vi "UI Example Subpanel.vi"(11 "CIF_UI in":refnum<class "CIF_UI.lvclass">) -> ()   [LabVIEW 2021, in "CIF Manager UI.lvlib"]
uses:
  CIF Manager UI.lvlib
  CIFUI/CIF_UI.lvclass
  CIFUI/Typedef/Core UI References.ctl
  CIFCore/Grpc/CIFCoreWrapper/CIFCoreWrapper.lvlib
panel:
  out "Current Config":string
  in  "New Config":string
  in  "Update Config":bool
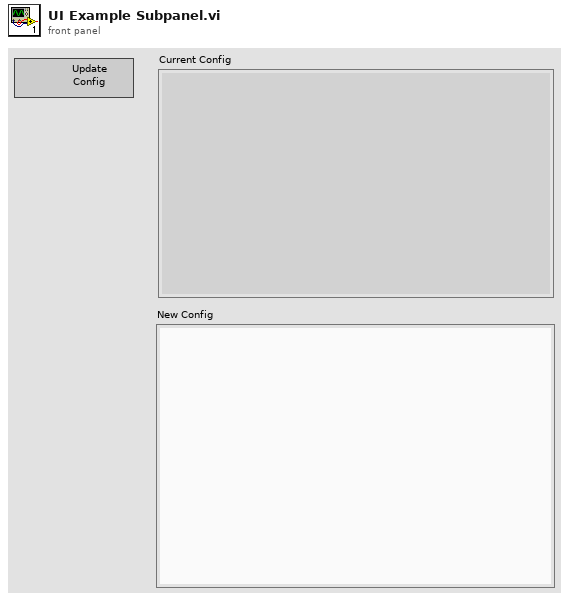
[diagram p1: front panel]
types:
  T1 = typedef "CIF_UI.lvclass/Core UI References.ctl" = cluster{"Discovered Plugins":refnum<vi>, "Discovered Plugins Valid":bool, "Loaded Plugins":refnum<vi>, "Loaded Plugins Valid":bool, "Publisher Channels":refnum<vi>, "Publisher Channels Valid":bool, "Subscriber Channels":refnum<vi>, "Subscriber Channels Valid":bool, "Plugin Status":refnum<vi>, "Plugin Status Valid":bool, "Channel Connection":refnum<vi>, "Channel Connection Valid":bool, "New Plugin Load":refnum<vi>, "New Plugin Load Valid":bool, "Errors":refnum<vi>, "Errors Valid":bool, "Plugin to Abort":refnum<vi>, "Plugin to Abort Valid":bool, "Connection":refnum<vi>, "Connection Valid":bool, "Exit":refnum<vi>, "Exit Valid":bool, "Run Listen":refnum<vi>, "Run Listen Valid":bool, "CIF Manager Tab":refnum<vi>, "Manger Tab Valid":bool, "Clear Local Error":refnum<vi>, "Clear Local Error Valid":bool, "Local Error":refnum<vi>, "Local Error Valid":bool, "System Errors":refnum<vi>, "System Errors Valid":bool, "Plugin Selection":refnum<vi>, "Plugin Selection Valid":bool}
  T2 = typedef "CIF_UI.lvclass/Plugin Connections.ctl" = cluster{"gRPC ID":T3, "Plugin Info":T4}
  T3 = typedef "grpc-lvsupport-release.lvlib/grpcId.ctl" = u64
  T4 = typedef "CIF_UI.lvclass/PluginInfo.ctl" = cluster{"Name":string, "Type":string, "grpc_port":i32, "Version":T5, "Node Status":T6}
  T5 = typedef "CIF_UI.lvclass/Version.ctl" = cluster{"Major":i32, "Minor":i32, "Fix":i32}
  T6 = typedef "CIFCoreCommon.lvlib/gRPC Reported Plugin Status.ctl" = cluster{"State":T7, "Timing Statistics (us)":T8, "FIFO Statistics (us)":T10, "error":T11, "Monitor Doubles":T12, "Monitor U64":T13, "Monitor I64":T14}
  T7 = typedef "CIFCoreCommon.lvlib/Plugin State.ctl" = enum32{"Null", "Creating", "Listening", "Running", "CleaningUp", "Destroying"}
  T8 = typedef "CIFCoreCommon.lvlib/Timing Statistics.ctl" = cluster{"Period":T9, "Wake Error":T9, "Execute":T9, "Housekeep":T9, "Idle":T9, "Cleanup":T9, "Custom 1 (custom units)":T9, "Custom 2 (custom units)":T9}
  T9 = typedef "CIFCoreCommon.lvlib/Timing Stats Base.ctl" = cluster{"Max":i64, "Avg":dbl, "Min":i64}
  T10 = typedef "CIFCoreCommon.lvlib/FIFO Statistics.ctl" = cluster{"From T0":T9, "From Previous Plugin":T9, "Output Error":T9}
  T11 = typedef "CIFCoreCommon.lvlib/Simple Error.ctl" = cluster{"status":bool, "code":i32}
  T12 = typedef "CIFCoreCommon.lvlib/Monitor Doubles.ctl" = cluster{"1":dbl, "2":dbl, "3":dbl, "4":dbl}
  T13 = typedef "CIFCoreCommon.lvlib/Monitor U64.ctl" = cluster{"1":u64, "2":u64, "3":u64, "4":u64}
  T14 = typedef "CIFCoreCommon.lvlib/Monitor I64.ctl" = cluster{"1":i64, "2":i64, "3":i64, "4":i64}
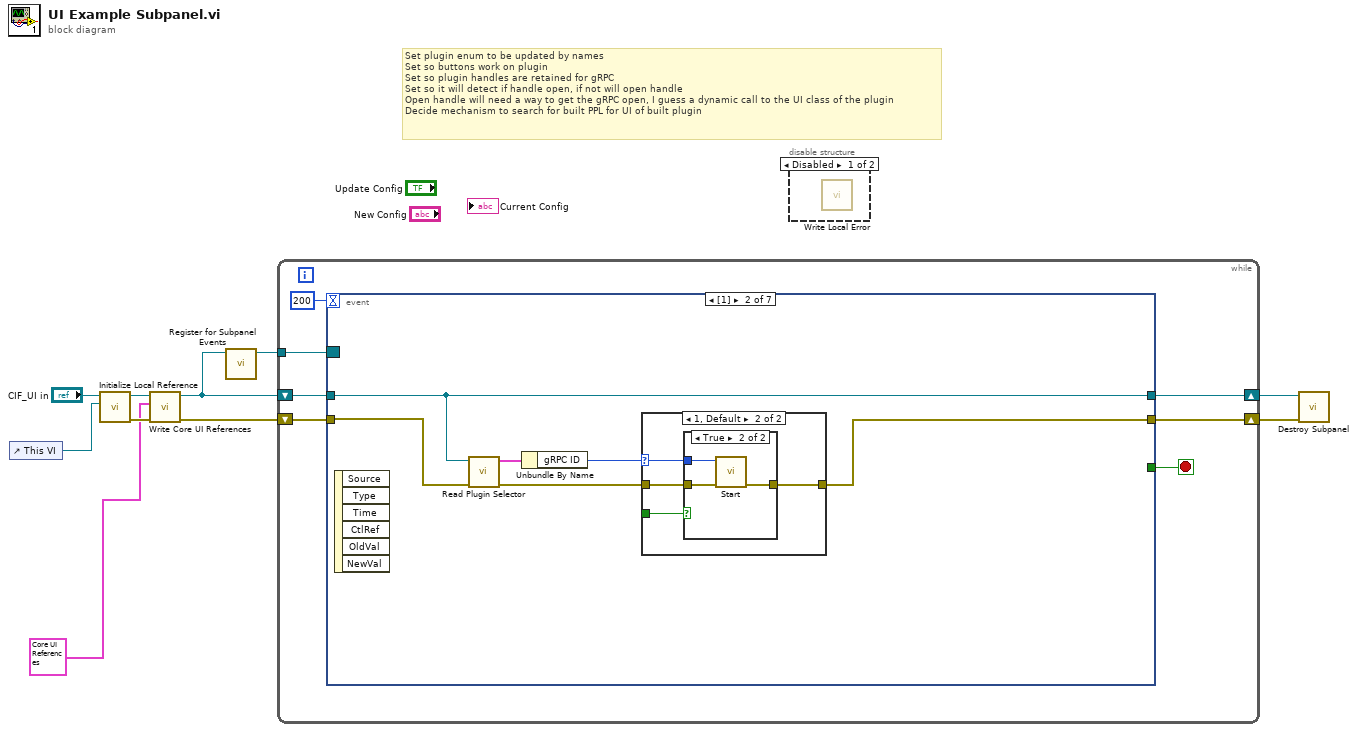
[diagram p0: block diagram]
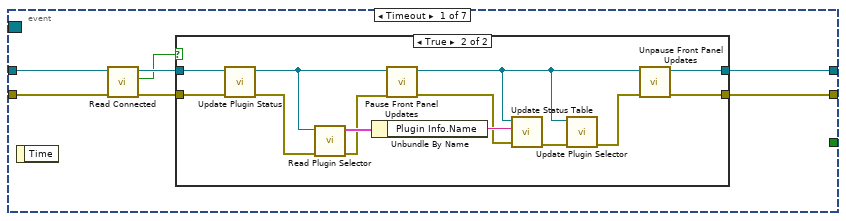
[diagram p3: hidden frame]
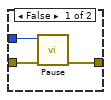
[diagram p6: hidden frame]
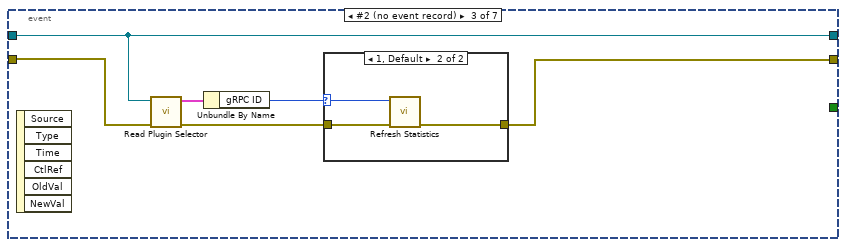
[diagram p7: hidden frame]
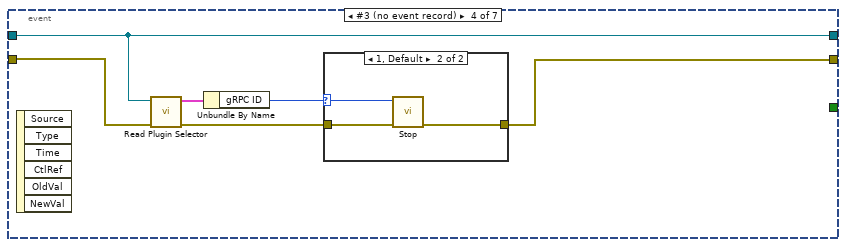
[diagram p9: hidden frame]
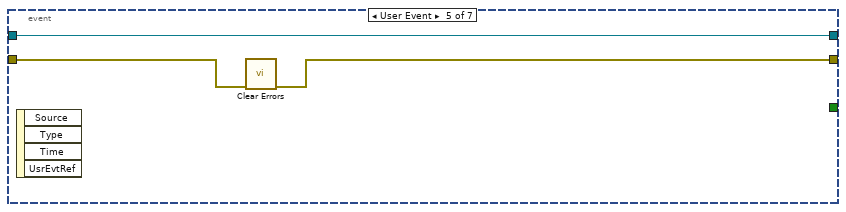
[diagram p11: hidden frame]
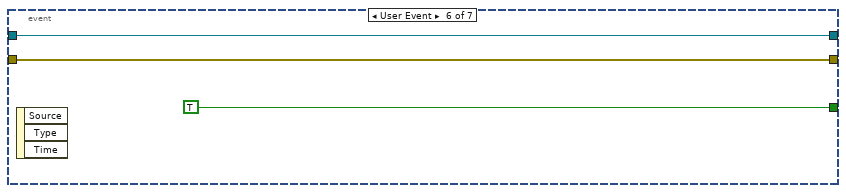
[diagram p12: hidden frame]
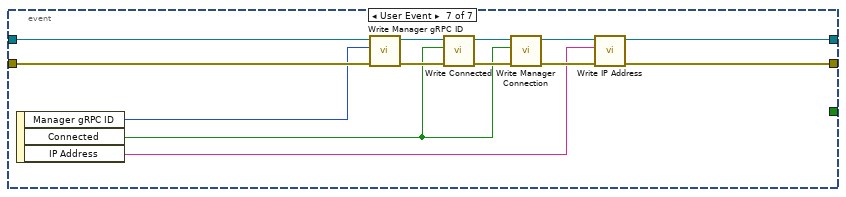
[diagram p13: hidden frame]
diagram:
  # "Set plugin enum to be updated by names\nSet so buttons work on plugin\nSet so plugin handles are retained for gRPC\nSet so it will detect if handle open, if not will open handle\nOpen handle will need a way to get the gRPC open, I guess a dynamic call to the UI class of the plugin\nDecide mechanism to search for built PPL for UI of built plugin"
  n1 = control-ref of="This VI"() -> (w7:refnum<vi>)
  n2 = call "Initialize Local Reference.vi"("This VI"=w7, "CIF_UI in"="CIF_UI in") -> ("error out"=w4:errorcluster, "CIF_UI out"=w5:refnum<class "CIF_UI.lvclass">)  [unwired: 8 in]
  n3 = call "Write Core UI References.vi"("error in (no error)"=w4, "UI References"=T1 {"Discovered Plugins"=refnum, "Discovered Plugins Valid"=FALSE, "Loaded Plugins"=refnum, "Loaded Plugins Valid"=FALSE, "Publisher Channels"=refnum, "Publisher Channels Valid"=FALSE, "Subscriber Channels"=refnum, "Subscriber Channels Valid"=FALSE, "Plugin Status"=refnum, "Plugin Status Valid"=FALSE, "Channel Connection"=refnum, "Channel Connection Valid"=FALSE, "New Plugin Load"=refnum, "New Plugin Load Valid"=FALSE, "Errors"=refnum, "Errors Valid"=FALSE, "Plugin to Abort"=refnum, "Plugin to Abort Valid"=FALSE, "Connection"=refnum, "Connection Valid"=FALSE, "Exit"=refnum, "Exit Valid"=FALSE, "Run Listen"=refnum, "Run Listen Valid"=FALSE, "CIF Manager Tab"=refnum, "Manger Tab Valid"=FALSE, "Clear Local Error"=refnum, "Clear Local Error Valid"=FALSE, "Local Error"=refnum, "Local Error Valid"=FALSE, "System Errors"=refnum, "System Errors Valid"=FALSE, "Plugin Selection"=refnum, "Plugin Selection Valid"=FALSE}, "CIF_UI in"=w5) -> ("error out"=w10:errorcluster, "CIF_UI out"=w9:refnum<class "CIF_UI.lvclass">)  [unwired: 7 in]
  n4 = call "Register for Subpanel Events.vi"("CIF_UI in"=w9) -> ("Event Registration Refnum"=w8:refnum<event-registration>)  [unwired: 9 in, 1 out]
  n5 = while {
    shift-right: [w12] -> w3
    shift-left: w9 -> [w15]
    shift-right: [w13] -> w2
    shift-left: w10 -> [w14]
    tunnel: w8 -> [w11]
    stop <- w16 stop-if-true
    n6 = event shown="[1]" {
      selector: w11 -> [_ _ _ _ _ _ _]
      dyn-events: _ -> [_ _ _ _ _ _ _]
      timeout: 200 -> [_ _ _ _ _ _ _]
      tunnel: [_ _ _ _ _ TRUE _] -> w16
      tunnel: w15 -> [w21 w40 w58 w68 w78 w82 w90]
      tunnel: w14 -> [w19 w46 w63 w73 w80 w81 w89]
      tunnel: [w18 w41 w59 w69 w79 w81 w87] -> w13
      tunnel: [w20 w40 w58 w68 w78 w82 w88] -> w12
      event Timeout {
        n7 = event-data() -> ()  [unwired: 1 in, 1 out]
        n8 = call "Read Connected.vi"("error in (no error)"=w19, "CIF_UI in"=w21) -> ("error out"=w23:errorcluster, "Connected"=w22:bool, "CIF_UI out"=w24:refnum<class "CIF_UI.lvclass">)  [unwired: 7 in]
        n9 = case shown="True" w22 {
          tunnel: w23 -> [w25 w37]
          tunnel: [w25 w39] -> w18
          tunnel: w24 -> [w26 w36]
          tunnel: [w26 w38] -> w20
          frame False {
          }
          frame True {
            n10 = call "Update Plugin Status.vi"("error in (no error)"=w37, "CIF_UI in"=w36) -> ("error out"=w33:errorcluster, "CIF_UI out"=w32:refnum<class "CIF_UI.lvclass">)  [unwired: 8 in]
            n11 = call "Read Plugin Selector.vi"("error in (no error)"=w33, "CIF_UI in"=w32) -> ("error out"=w31:errorcluster, "Plugin Info"=w35:T2)  [unwired: 8 in]
            n12 = Unbundle By Name(w35) -> ("Plugin Info.Name"=w34:string)
            n13 = call "Pause Front Panel Updates.vi"("error in (no error)"=w31, "CIF_UI in"=w32) -> ("error out"=w30:errorcluster, "CIF_UI out"=w28:refnum<class "CIF_UI.lvclass">)  [unwired: 8 in]
            n14 = call "Update Status Table.vi"("error in (no error)"=w30, "Plugin Filter"=w34, "CIFManager_UI in"=w28) -> ("error out"=w29:errorcluster)  [unwired: 8 in]
            n15 = call "Update Plugin Selector.vi"("error in (no error)"=w29, "CIF_UI in"=w28) -> ("error out"=w27:errorcluster)  [unwired: 9 in]
            n16 = call "Unpause Front Panel Updates.vi"("error in (no error)"=w27, "CIF_UI in"=w28) -> ("error out"=w39:errorcluster, "CIF_UI out"=w38:refnum<class "CIF_UI.lvclass">)  [unwired: 8 in]
          }
        }
      }
      event #1 (no event record) {
        n17 = event-data() -> ()  [unwired: 1 in, 6 out]
        n18 = call "Read Plugin Selector.vi"("error in (no error)"=w46, "CIF_UI in"=w40) -> ("error out"=w43:errorcluster, "Plugin Info"=w45:T2)  [unwired: 8 in]
        n19 = Unbundle By Name(w45) -> ("gRPC ID"=w44:T3)
        n20 = case shown="1, Default" w44 {
          selector: w44 -> [_ w51]
          tunnel: w43 -> [w47 w50]
          tunnel: [_ w49] -> w42
          tunnel: [w47 w48] -> w41
          frame 0 {
          }
          frame 1, Default {
            n21 = case shown="True" w49 {
              tunnel: w51 -> [w54 w57]
              tunnel: w50 -> [w53 w56]
              tunnel: [w52 w55] -> w48
              frame False {
                n22 = call "Pause.vi"("error in"=w53, "gRPC ID"=w54) -> ("error out"=w52:errorcluster)  [unwired: 8 in, 1 out]
              }
              frame True {
                n23 = call "Start.vi"("error in"=w56, "gRPC ID"=w57) -> ("error out"=w55:errorcluster)  [unwired: 8 in, 1 out]
              }
            }
          }
        }
      }
      event #2 (no event record) {
        n24 = event-data() -> ()  [unwired: 1 in, 6 out]
        n25 = call "Read Plugin Selector.vi"("error in (no error)"=w63, "CIF_UI in"=w58) -> ("error out"=w60:errorcluster, "Plugin Info"=w62:T2)  [unwired: 8 in]
        n26 = Unbundle By Name(w62) -> ("gRPC ID"=w61:T3)
        n27 = case shown="1, Default" w61 {
          selector: w61 -> [_ w67]
          tunnel: w60 -> [w64 w66]
          tunnel: [w64 w65] -> w59
          frame 0 {
          }
          frame 1, Default {
            n28 = call "Refresh Statistics.vi"("error in"=w66, "gRPC ID"=w67) -> ("error out"=w65:errorcluster)  [unwired: 8 in, 1 out]
          }
        }
      }
      event #3 (no event record) {
        n29 = event-data() -> ()  [unwired: 1 in, 6 out]
        n30 = call "Read Plugin Selector.vi"("error in (no error)"=w73, "CIF_UI in"=w68) -> ("error out"=w70:errorcluster, "Plugin Info"=w72:T2)  [unwired: 8 in]
        n31 = Unbundle By Name(w72) -> ("gRPC ID"=w71:T3)
        n32 = case shown="1, Default" w71 {
          selector: w71 -> [_ w75]
          tunnel: w70 -> [w74 w77]
          tunnel: [w74 w76] -> w69
          frame 0 {
          }
          frame 1, Default {
            n33 = call "Stop.vi"("error in"=w77, "gRPC ID"=w75) -> ("error out"=w76:errorcluster)  [unwired: 8 in, 1 out]
          }
        }
      }
      event User Event {
        n34 = event-data() -> ()  [unwired: 1 in, 4 out]
        n35 = call <vilib>:"Clear Errors.vi"("error in (no error)"=w80) -> ("error out"=w79:errorcluster)  [unwired: 5 in, 1 out]
      }
      event User Event {
        n36 = event-data() -> ()  [unwired: 1 in, 3 out]
      }
      event User Event {
        n37 = event-data() -> ("Manager gRPC ID"=w84:T3, "Connected"=w85:bool, "IP Address"=w86:string)  [unwired: 1 in]
        n38 = call "Write Manager gRPC ID.vi"("error in (no error)"=w89, "gRPCid"=w84, "CIF_UI in"=w90) -> ("error out"=w95:errorcluster, "CIF_UI out"=w96:refnum<class "CIF_UI.lvclass">)  [unwired: 7 in]
        n39 = call "Write Connected.vi"("error in (no error)"=w95, "Connected"=w85, "CIF_UI in"=w96) -> ("error out"=w93:errorcluster, "CIF_UI out"=w94:refnum<class "CIF_UI.lvclass">)  [unwired: 7 in]
        n40 = call "Write Manager Connection.vi"("error in (no error)"=w93, "Manager Connection"=w85, "CIF_UI in"=w94) -> ("error out"=w91:errorcluster, "CIF_UI out"=w92:refnum<class "CIF_UI.lvclass">)  [unwired: 7 in]
        n41 = call "Write IP Address.vi"("error in (no error)"=w91, "IP Address"=w86, "CIF_UI in"=w92) -> ("error out"=w87:errorcluster, "CIF_UI out"=w88:refnum<class "CIF_UI.lvclass">)  [unwired: 7 in]
      }
    }
  }
  n42 = disable-structure shown="Disabled" {
    frame Disabled {
      n43 = call "Write Local Error.vi"() -> ()  [unwired: 11 in, 1 out]
    }
    frame Enabled {
    }
  }
  n44 = call "Destroy Subpanel.vi"("error in (no error)"=w2, "CIF_UI in"=w3) -> ()  [unwired: 8 in, 2 out]
